vi "HexToFloat.vi"(11 "数组":u16[](array[numeric]) format="%04xH") -> (3 "FLOAT":sgl[](array[numeric]))   [LabVIEW 2022 SP3, in "挥发酚.lvlib"]
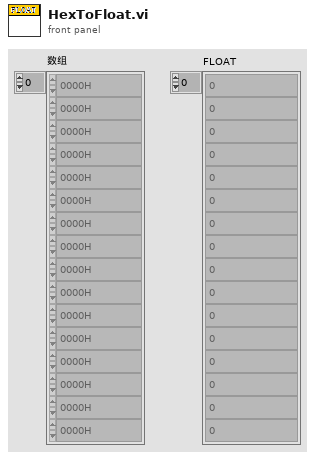
[diagram p1: front panel]
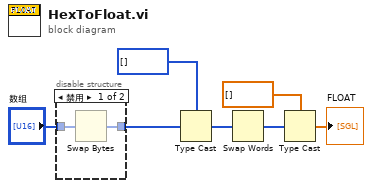
[diagram p0: block diagram]
diagram:
  n1 = disable-structure shown="禁用" {
    disable-tunnel: "数组" -> [w9 w10]
    disable-tunnel: [w8 w10] -> w1
    frame Disabled {
      n2 = Swap Bytes(anything=w9) -> (byte swapped=w8:u16[])
    }
    frame Enabled {
    }
  }
  n3 = Type Cast(type=u32[] [], x=w1) -> (*(type *) &x=w4:u32[])
  n4 = Swap Words(1:w4) -> (0:w3:u32[])
  n5 = Type Cast(type=sgl[] [], x=w3) -> (*(type *) &x=→"FLOAT":sgl[])
